vi "G#Object_GetAllObjects.vi"(1 "full class name (\"\")":string, 2 "only refs (F)":bool, 5 "error in (no error)":errorcluster) -> (10 "all objects":T1[](array[typedef]), 12 "all refs":refnum<class "G#Object.lvclass">[](array[class]), 15 "class information":T3[](array[typedef]), 19 "error out":errorcluster)   [LabVIEW 2020, in "G#Object.lvclass"]
doc: "Returns all objects of the specified class. If \"full class name\" is empty, all objects of all classes will be returned."
uses:
  <vilib>/addons/_AddQ/G#Object/G#Object.lvclass
  <vilib>/addons/_AddQ/G#Object/utils/G#Object_ClassInfoType.ctl
  <vilib>/addons/_AddQ/G#Object/utils/G#Object_ObjectInfoType.ctl
  <vilib>/addons/_AddQ/G#Object/utils/G#Object_CreateMethod.ctl
  <vilib>/addons/_AddQ/G#Object/G#Object.lvclass/G#Object.ctl
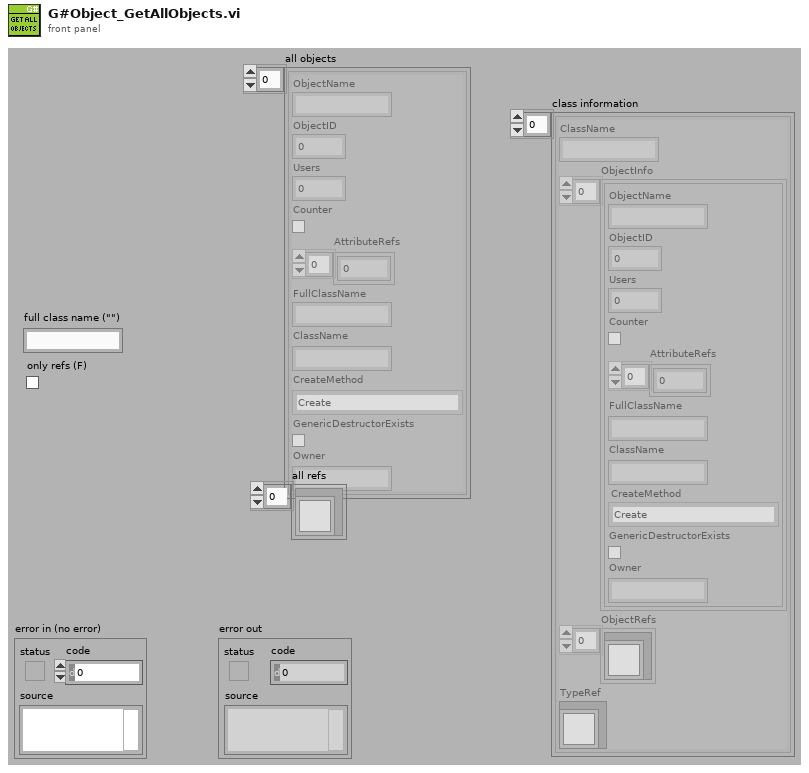
[diagram p1: front panel]
types:
  T1 = typedef "G#Object.lvclass/G#Object_ObjectInfoType.ctl" = cluster{"ObjectName":string, "ObjectID":u32, "Users":i32, "Counter":bool, "AttributeRefs":u32[], "FullClassName":string, "ClassName":string, "CreateMethod":T2, "GenericDestructorExists":bool, "Owner":string}
  T2 = typedef "G#Object.lvclass/G#Object_CreateMethod.ctl" = enum16{"Create", "Create or look up existing", "Look up existing"}
  T3 = typedef "G#Object.lvclass/G#Object_ClassInfoType.ctl" = cluster{"ClassName":string, "ObjectInfo":T1[], "ObjectRefs":refnum<class "G#Object.lvclass">[], "TypeRef":refnum<class "G#Object.lvclass">}
  T4 = cluster{"full class name (\"\")":string, "Ref":refnum<class "G#Object.lvclass">}
  T5 = cluster{"full class name (\"\")":string, "Ref":refnum<class "G#Object.lvclass">}[]
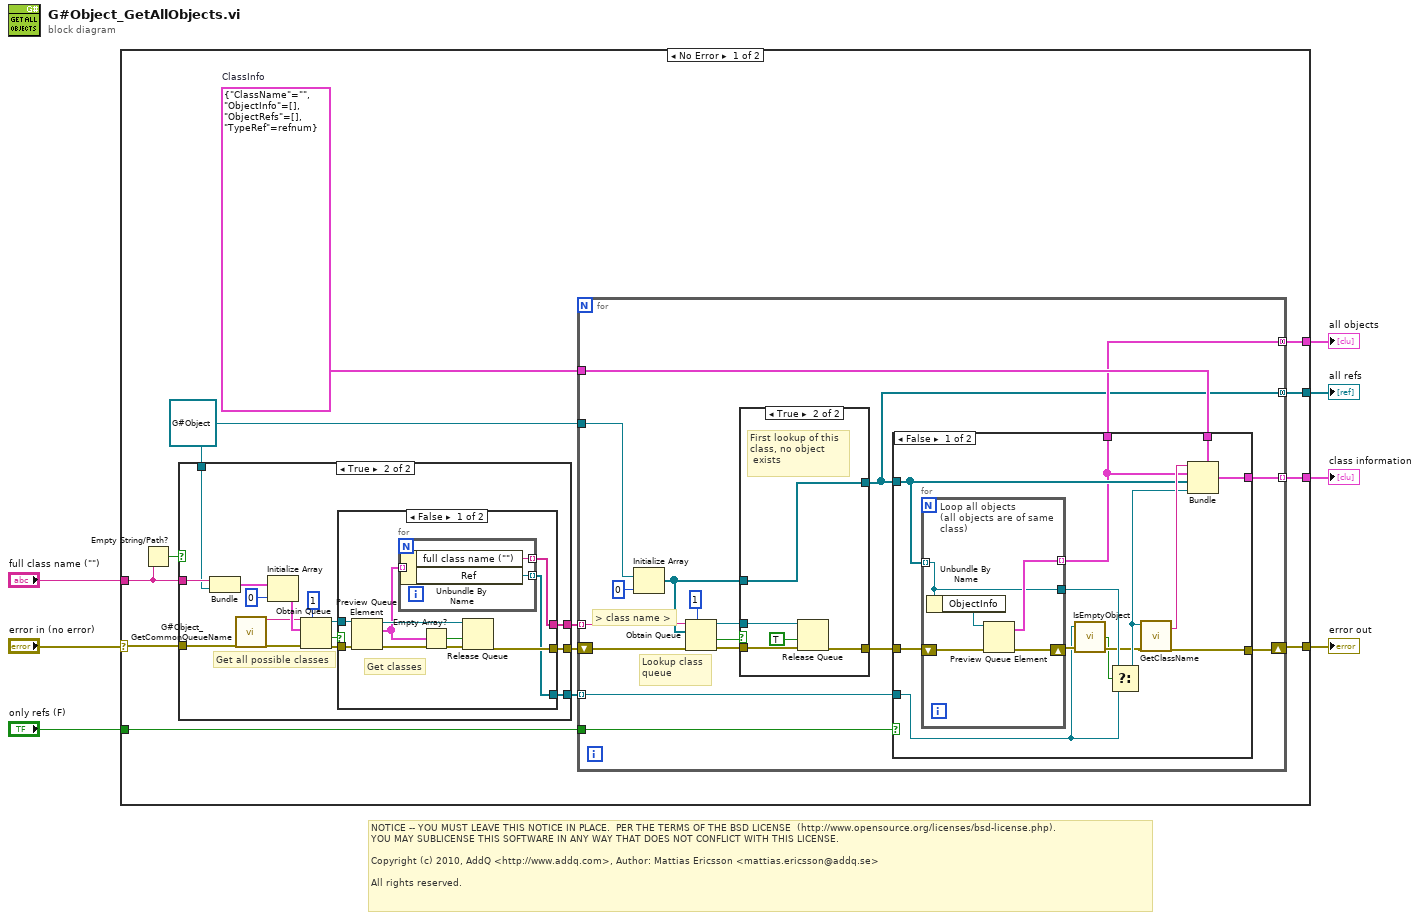
[diagram p0: block diagram]
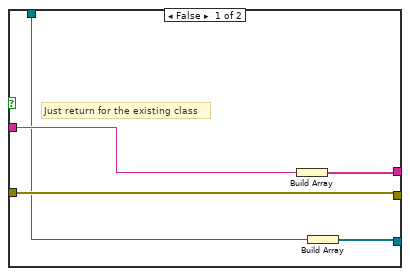
[diagram p2: hidden frame]
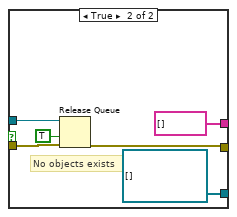
[diagram p3: hidden frame]
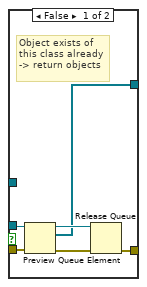
[diagram p5: hidden frame]
diagram:
  # "NOTICE -- YOU MUST LEAVE THIS NOTICE IN PLACE.  PER THE TERMS OF THE BSD LICENSE  (http://www.opensource.org/licenses/bsd-license.php).\nYOU MAY SUBLICENSE THIS SOFTWARE IN ANY WAY THAT DOES NOT CONFLICT WITH THIS LICENSE.\n\nCopyright (c) 2010, AddQ <http://www.addq.com>, Author: Mattias Ericsson <mattias.ericsson@addq.se>\n\nAll rights reserved."
  n1 = case shown="No Error" "error in (no error)" {
    selector: "error in (no error)" -> [w17 w106]
    tunnel: [w15 w106] -> w6
    tunnel: [w8 _] -> w5
    tunnel: [w16 _] -> w4
    tunnel: [w9 _] -> w3
    tunnel: "only refs (F)" -> [w14 _]
    tunnel: "full class name (\"\")" -> [w12 _]
    frame No Error {
      w11 = refnum<class "G#Object.lvclass"> refnum ("Ref")
      w18 = T3 {"ClassName"="", "ObjectInfo"=[], "ObjectRefs"=[], "TypeRef"=refnum}  # ClassInfo
      n2 = Empty String/Path?(string/path=w12) -> (empty?=w13:bool)
      n3 = case shown="True" w13 {
        tunnel: [w24 w34] -> w20
        tunnel: [w25 w33] -> w19
        tunnel: w17 -> [w25 w28]
        tunnel: w12 -> [w23 w31]
        tunnel: w11 -> [w22 w29]
        tunnel: [w21 w30] -> w10
        frame False {
          # "Just return for the existing class"
          n4 = Build Array(w23) -> (w24:string[])
          n5 = Build Array(w22) -> (w21:refnum<class "G#Object.lvclass">[])
        }
        frame True {
          # "Get all possible classes"
          n6 = Bundle("full class name (\"\")"=w31, "Ref"=w29) -> (w32:T4)  [unwired: 1 in]
          n7 = call <vilib>:"G#Object_GetCommonQueueName.vi"("error in (no error)"=w28) -> ("queue name"=w26:string, "error out"=w27:errorcluster)  [unwired: 17 in]
          n8 = Initialize Array(w32, 0 ("dimension size")) -> (w35:T5)
          n9 = Obtain Queue(max queue size (-1, unlimited)=1, name (unnamed)=w26, element data type=w35, error in (no error)=w27) -> (queue out=w38:refnum<queue>, created new?=w40:bool, error out=w39:errorcluster)  [unwired: 1 in]
          n10 = case shown="False" w40 {
            tunnel: w39 -> [w49 w55]
            tunnel: w38 -> [w48 w56]
            tunnel: [w44 string[] []] -> w34
            tunnel: [w47 w58] -> w33
            tunnel: [w43 refnum<class "G#Object.lvclass">[] []] -> w30
            frame False {
              # "Get classes"
              n11 = Preview Queue Element(queue=w48, error in (no error)=w49) -> (queue out=w45:refnum<queue>, element=w42:T5, error out=w46:errorcluster)  [unwired: 1 in, 1 out]
              n12 = for {
                tunnel: [w52] -> w44 mode=indexing
                tunnel: w42 -> [w51] mode=indexing
                tunnel: [w50] -> w43 mode=indexing
                n13 = Unbundle By Name(w51) -> ("full class name (\"\")"=w52:string, "Ref"=w50:refnum<class "G#Object.lvclass">)
              }
              n14 = Empty Array?(array=w42) -> (empty?=w41:bool)
              n15 = Release Queue(queue=w45, force destroy? (F)=w41, error in (no error)=w46) -> (error out=w47:errorcluster)  [unwired: 2 out]
            }
            frame True {
              # "No objects exists"
              n16 = Release Queue(queue=w56, force destroy? (F)=TRUE, error in (no error)=w55) -> (error out=w58:errorcluster)  [unwired: 2 out]
            }
          }
        }
      }
      n17 = for {
        shift-right: [w67] -> w15
        shift-left: w19 -> [w71]
        tunnel: w20 -> [w65] mode=indexing
        tunnel: [w70] -> w16 mode=indexing
        tunnel: w11 -> [w64]
        tunnel: w18 -> [w69]
        tunnel: w14 -> [w66]
        tunnel: w10 -> [w61] mode=indexing
        tunnel: [w60] -> w9 mode=concatenating
        tunnel: [w59] -> w8 mode=concatenating
        # "Loop all classes"
        # "> class name >"
        # "Lookup class\nqueue"
        n18 = Initialize Array(w64, 0 ("dimension size")) -> (w63:refnum<class "G#Object.lvclass">[])
        n19 = Obtain Queue(max queue size (-1, unlimited)=1, name (unnamed)=w65, element data type=w63, error in (no error)=w71) -> (queue out=w72:refnum<queue>, created new?=w73:bool, error out=w74:errorcluster)  [unwired: 1 in]
        n20 = case shown="True" w73 {
          tunnel: w74 -> [w99 w101]
          tunnel: w72 -> [w98 w102]
          tunnel: w63 -> [_ w105]
          tunnel: [w100 w104] -> w68
          tunnel: [w95 w105] -> w59
          frame False {
            # "Object exists of\nthis class already\n-> return objects"
            n21 = Preview Queue Element(queue=w98, error in (no error)=w99) -> (queue out=w96:refnum<queue>, element=w95:refnum<class "G#Object.lvclass">[], error out=w97:errorcluster)  [unwired: 1 in, 1 out]
            n22 = Release Queue(queue=w96, error in (no error)=w97) -> (error out=w100:errorcluster)  [unwired: 1 in, 2 out]
          }
          frame True {
            # "First lookup of this\nclass, no object\n exists"
            n23 = Release Queue(queue=w102, force destroy? (F)=TRUE, error in (no error)=w101) -> (error out=w104:errorcluster)  [unwired: 2 out]
          }
        }
        n24 = case shown="False" w66 {
          tunnel: [w88 _] -> w70
          tunnel: w69 -> [w87 _]
          tunnel: w68 -> [w86 w94]
          tunnel: w59 -> [w77 _]
          tunnel: [w85 w94] -> w67
          tunnel: [w76 _] -> w60
          tunnel: w61 -> [w79 _]
          frame False {
            n25 = for {
              shift-right: [w92] -> w81
              shift-left: w86 -> [w93]
              tunnel: w77 -> [w89] mode=indexing
              tunnel: [w90] -> w76 mode=indexing
              tunnel: [w89] -> w83
              # "Loop all objects\n(all objects are of same\nclass)"
              n26 = Unbundle By Name(w89) -> ("ObjectInfo"=w91:refnum<queue>)
              n27 = Preview Queue Element(queue=w91, error in (no error)=w93) -> (element=w90:T1, error out=w92:errorcluster)  [unwired: 1 in, 2 out]
            }
            n28 = call-dynamic "IsEmptyObject.vi"("error in (no error)"=w81, "reference in"=w79) -> ("error out"=w80:errorcluster, "is empty?"=w78:bool)  [unwired: 1 in, 1 out]
            n29 = Select(t=w83, s=w78, f=w79) -> (s? t:f=w82:refnum<class "G#Object.lvclass">)
            n30 = call-dynamic "GetClassName.vi"("reference in"=w82, "error in (no error)"=w80) -> ("class name"=w84:string, "error out"=w85:errorcluster)  [unwired: 13 in, 3 out]
            n31 = Bundle(cluster=w87, "ClassName"=w84, "ObjectInfo"=w76, "ObjectRefs"=w77, "TypeRef"=w82) -> (w88:T3)
          }
          frame True {
            # "Only refs are wanted, skip object info"
          }
        }
      }
    }
    frame Error {
    }
  }
  "error out" <- w6
  "class information" <- w4
  "all objects" <- w3
  "all refs" <- w5
